vi "GetType.vi"(8 "error in (no error)":errorcluster, 11 "Configure RangeMin Msg":refnum<class "Configure RangeMin Msg.lvclass">) -> (0 "error out":errorcluster, 2 "Data Sample":variant, 3 "Configure RangeMin Msg":refnum<class "Configure RangeMin Msg.lvclass">)   [LabVIEW 2015, in "CS++Motor.lvlib" / "Configure RangeMin Msg.lvclass"]
uses:
  Configure RangeMin Msg.lvclass
  Configure RangeMin Msg.lvclass/Configure RangeMin Msg.ctl
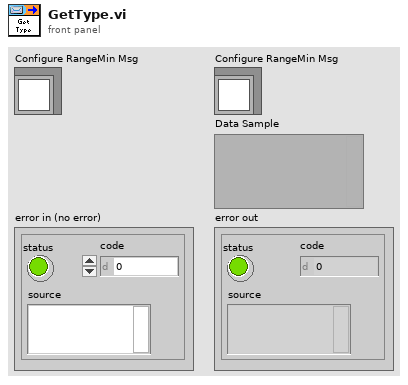
[diagram p1: front panel]
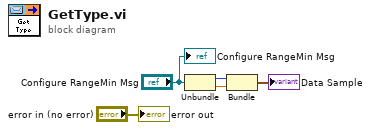
[diagram p0: block diagram]
diagram:
  n1 = Unbundle("Configure RangeMin Msg") -> (w2:u8, w1:dbl)
  n2 = Bundle("AxisNumber"=w2, "RangeMin"=w1) -> (→"Data Sample":cluster{"AxisNumber":u8, "RangeMin":dbl})  [unwired: 1 in]
  "error out" <- "error in (no error)"
  "Configure RangeMin Msg" <- "Configure RangeMin Msg"
